vi "TS Engine Shutdown.vi"(8 "error in (no error)":errorcluster, 11 "Auto UI in":refnum<class "Auto UI.lvclass">) -> (0 "error out":errorcluster, 2 "Shutdown":bool, 3 "Auto UI out":refnum<class "Auto UI.lvclass">)   [LabVIEW 2023, in "GUI.lvlib" / "Auto UI.lvlib" / "Auto UI.lvclass"]
uses:
  Auto UI.lvclass
  Auto UI.lvclass/Auto UI.ctl
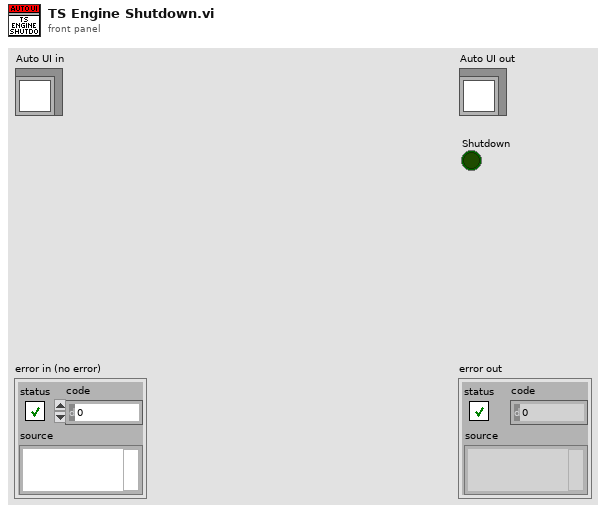
[diagram p1: front panel]
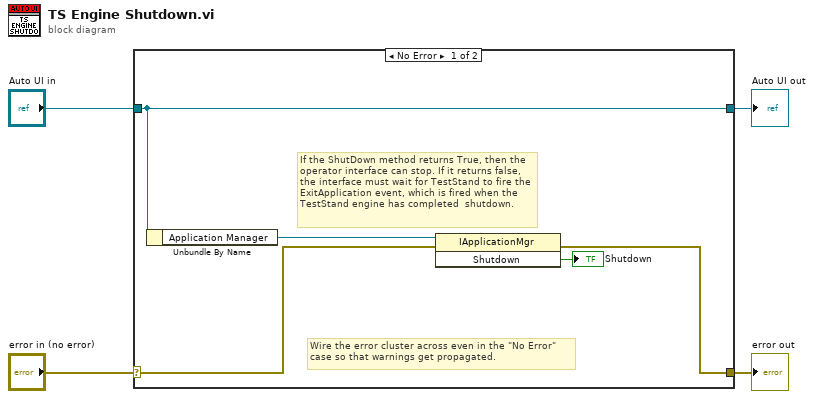
[diagram p0: block diagram]
diagram:
  n1 = case shown="No Error" "error in (no error)" {
    selector: "error in (no error)" -> [w7 w11]
    tunnel: [w6 w11] -> w3
    tunnel: [w9 w10] -> w1
    tunnel: "Auto UI in" -> [w9 w10]
    frame No Error {
      # "If the ShutDown method returns True, then the operator interface can stop. If it returns false, the interface must wait for TestStand to fire the ExitApplication event, which is fired when the TestStand engine has completed  shutdown."
      # "Wire the error cluster across even in the \"No Error\"\ncase so that warnings get propagated."
      n2 = Unbundle By Name(w9) -> ("Application Manager"=w8:refnum<k7>)
      n3 = invoke class="IApplicationMgr" method="Shutdown"(reference=w8, error in=w7) -> (error out=w6:errorcluster, "Shutdown"=→"Shutdown":bool)  [unwired: 1 in, 1 out]
    }
    frame Error {
    }
  }
  "error out" <- w3
  "Auto UI out" <- w1
